vi "TEST_NT_HELPER_BOOL.vi"() -> ()   [LabVIEW 2023]
uses:
  <vilib>/Rock Robotics/Network Tables/NT Read Boolean.vi
  <vilib>/Rock Robotics/Network Tables/NT Write Boolean.vi
panel:
  out "value 2":bool
  out "value":bool
  in  "name 2":string="Test4150Val1b"
  in  "name":string="Test4150Val2b"
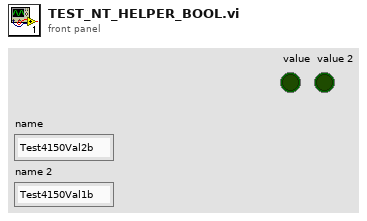
[diagram p1: front panel]
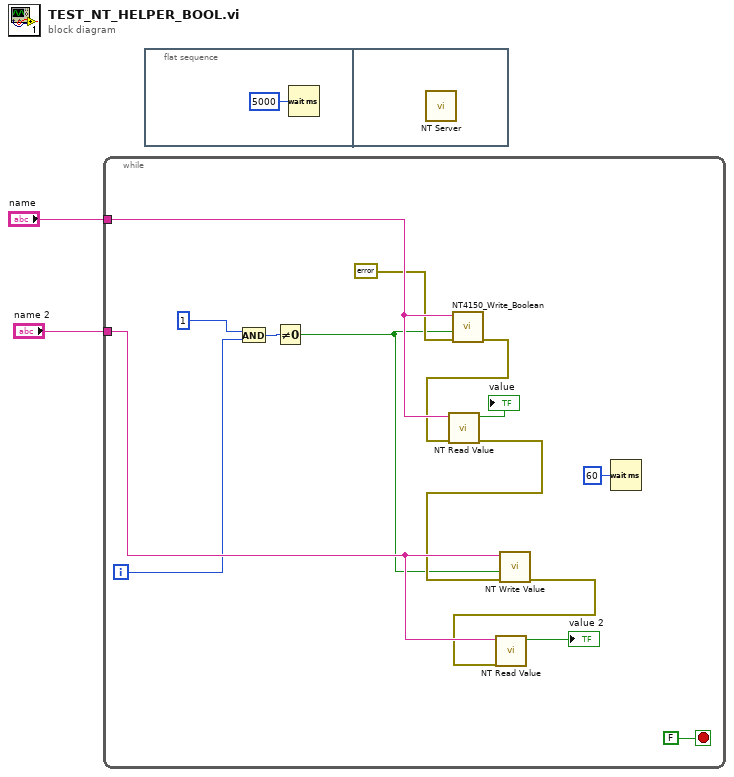
[diagram p0: block diagram]
diagram:
  n1 = while {
    tunnel: "name" -> [w16]
    tunnel: "name 2" -> [w14]
    i -> [w8]
    stop <- FALSE stop-if-true
    n2 = And(x=1, y=w8) -> (x .and. y?=w7:i32)
    n3 = Not Equal To 0?(x=w7) -> (x != 0?=w6:bool)
    n4 = call "NT4150_Write_Boolean.vi"("error in"=errorcluster {"status"=FALSE, "code"=0, "source"=""}, "value"=w6, "name"=w16) -> ("error out"=w13:errorcluster)  [unwired: 8 in]
    n5 = call-poly <vilib>:"NT Read Value.vi"("error in"=w13, "name"=w16) -> ("error out"=w12:errorcluster, "value"=→"value":bool)  [unwired: 7 in, 1 out]
    n6 = call-poly <vilib>:"NT Write Value.vi"("error in"=w12, "value"=w6, "name"=w14) -> ("error out"=w11:errorcluster)  [unwired: 8 in]
    n7 = call-poly <vilib>:"NT Read Value.vi"("error in"=w11, "name"=w14) -> ("value"=→"value 2":bool)  [unwired: 7 in, 2 out]
    n8 = Wait (ms)(milliseconds to wait=u32 60) -> ()  [unwired: 1 out]
  }
  n9 = flat-sequence {
    frame #0 {
      n10 = Wait (ms)(milliseconds to wait=u32 5000) -> ()  [unwired: 1 out]
    }
    frame #1 {
      n11 = call <vilib>:"NT Server.vi"() -> ()  [unwired: 11 in, 1 out]
    }
  }
